vi "FGV Grenzwerte PNS.vi"(0 "Grenzwerte PNS":T5={"Filter:"={"Sollwert"=0.0, "Warn-Min"=0.0, "Warn-Max"=0.0, "Abschalt-Min"=0.0, "Abschalt-Max"=0.0, "Regler"=1, "AnlagenParameter"=""}, "Ventilplatte:"={"Sollwert"=0.0, "Warn-Min"=0.0, "Warn-Max"=0.0, "Abschalt-Min"=0.0, "Abschalt-Max"=0.0, "Regler"=1, "AnlagenParameter"=""}, "Heizleitung 1:"={"Sollwert"=0.0, "Warn-Min"=0.0, "Warn-Max"=0.0, "Abschalt-Min"=0.0, "Abschalt-Max"=0.0, "Regler"=1, "AnlagenParameter"=""}, "Heizleitung 2:"={"Sollwert"=0.0, "Warn-Min"=0.0, "Warn-Max"=0.0, "Abschalt-Min"=0.0, "Abschalt-Max"=0.0, "Regler"=1, "AnlagenParameter"=""}, "Heizleitung 3:"={"Sollwert"=0.0, "Warn-Min"=0.0, "Warn-Max"=0.0, "Abschalt-Min"=0.0, "Abschalt-Max"=0.0, "Regler"=1, "AnlagenParameter"=""}, "Heizleitung 4:"={"Sollwert"=0.0, "Warn-Min"=0.0, "Warn-Max"=0.0, "Abschalt-Min"=0.0, "Abschalt-Max"=0.0, "Regler"=1, "AnlagenParameter"=""}, "Heizleitung 5:"={"Sollwert"=0.0, "Warn-Min"=0.0, "Warn-Max"=0.0, "Abschalt-Min"=0.0, "Abschalt-Max"=0.0, "Regler"=1, "AnlagenParameter"=""}, "Heizleitung 6:"={"Sollwert"=0.0, "Warn-Min"=0.0, "Warn-Max"=0.0, "Abschalt-Min"=0.0, "Abschalt-Max"=0.0, "Regler"=1, "AnlagenParameter"=""}} {"Heizleitung 6:"."Regler" items=["aktiv", "inaktiv"]; "Heizleitung 6:"."Abschalt-Max" format="%#_5g"; "Heizleitung 6:"."Abschalt-Min" format="%#_5g"; "Heizleitung 6:"."Warn-Max" format="%#_5g"; "Heizleitung 6:"."Warn-Min" format="%#_5g"; "Heizleitung 6:"."Sollwert" format="%#_5g"; "Heizleitung 5:"."Regler" items=["aktiv", "inaktiv"]; "Heizleitung 5:"."Abschalt-Max" format="%#_5g"; "Heizleitung 5:"."Abschalt-Min" format="%#_5g"; "Heizleitung 5:"."Warn-Max" format="%#_5g"; "Heizleitung 5:"."Warn-Min" format="%#_5g"; "Heizleitung 5:"."Sollwert" format="%#_5g"; "Heizleitung 4:"."Regler" items=["aktiv", "inaktiv"]; "Heizleitung 4:"."Abschalt-Max" format="%#_5g"; "Heizleitung 4:"."Abschalt-Min" format="%#_5g"; "Heizleitung 4:"."Warn-Max" format="%#_5g"; "Heizleitung 4:"."Warn-Min" format="%#_5g"; "Heizleitung 4:"."Sollwert" format="%#_5g"; "Heizleitung 3:"."Regler" items=["aktiv", "inaktiv"]; "Heizleitung 3:"."Abschalt-Max" format="%#_5g"; "Heizleitung 3:"."Abschalt-Min" format="%#_5g"; "Heizleitung 3:"."Warn-Max" format="%#_5g"; "Heizleitung 3:"."Warn-Min" format="%#_5g"; "Heizleitung 3:"."Sollwert" format="%#_5g"; "Heizleitung 2:"."Regler" items=["aktiv", "inaktiv"]; "Heizleitung 2:"."Abschalt-Max" format="%#_5g"; "Heizleitung 2:"."Abschalt-Min" format="%#_5g"; "Heizleitung 2:"."Warn-Max" format="%#_5g"; "Heizleitung 2:"."Warn-Min" format="%#_5g"; "Heizleitung 2:"."Sollwert" format="%#_5g"; "Heizleitung 1:"."Regler" items=["aktiv", "inaktiv"]; "Heizleitung 1:"."Abschalt-Max" format="%#_5g"; "Heizleitung 1:"."Abschalt-Min" format="%#_5g"; "Heizleitung 1:"."Warn-Max" format="%#_5g"; "Heizleitung 1:"."Warn-Min" format="%#_5g"; "Heizleitung 1:"."Sollwert" format="%#_5g"; "Ventilplatte:"."Regler" items=["aktiv", "inaktiv"]; "Ventilplatte:"."Abschalt-Max" format="%#_5g"; "Ventilplatte:"."Abschalt-Min" format="%#_5g"; "Ventilplatte:"."Warn-Max" format="%#_5g"; "Ventilplatte:"."Warn-Min" format="%#_5g"; "Ventilplatte:"."Sollwert" format="%#_5g"; "Filter:"."Regler" items=["aktiv", "inaktiv"]; "Filter:"."Abschalt-Max" format="%#_5g"; "Filter:"."Abschalt-Min" format="%#_5g"; "Filter:"."Warn-Max" format="%#_5g"; "Filter:"."Warn-Min" format="%#_5g"; "Filter:"."Sollwert" format="%#_5g"}, 1 "T90":bool, 2 "T90 lüften":bool, 5 "IP-Adresse":string, 7 "Anweisungscode":u16, 9 "Zustand":T1, 11 "Samplepoint":u16=1, 12 "Aktionen FGV Grenzwerte":T7) -> (4 "Grenzwerte PNS 2":T2={"Filter:"={"Sollwert"=0.0, "Warn-Min"=0.0, "Warn-Max"=0.0, "Abschalt-Min"=0.0, "Abschalt-Max"=0.0, "Regler"=1, "AnlagenParameter"=""}, "Ventilplatte:"={"Sollwert"=0.0, "Warn-Min"=0.0, "Warn-Max"=0.0, "Abschalt-Min"=0.0, "Abschalt-Max"=0.0, "Regler"=1, "AnlagenParameter"=""}, "Heizleitung 1:"={"Sollwert"=0.0, "Warn-Min"=0.0, "Warn-Max"=0.0, "Abschalt-Min"=0.0, "Abschalt-Max"=0.0, "Regler"=1, "AnlagenParameter"=""}, "Heizleitung 2:"={"Sollwert"=0.0, "Warn-Min"=0.0, "Warn-Max"=0.0, "Abschalt-Min"=0.0, "Abschalt-Max"=0.0, "Regler"=1, "AnlagenParameter"=""}, "Heizleitung 3:"={"Sollwert"=0.0, "Warn-Min"=0.0, "Warn-Max"=0.0, "Abschalt-Min"=0.0, "Abschalt-Max"=0.0, "Regler"=1, "AnlagenParameter"=""}, "Heizleitung 4:"={"Sollwert"=0.0, "Warn-Min"=0.0, "Warn-Max"=0.0, "Abschalt-Min"=0.0, "Abschalt-Max"=0.0, "Regler"=1, "AnlagenParameter"=""}, "Heizleitung 5:"={"Sollwert"=0.0, "Warn-Min"=0.0, "Warn-Max"=0.0, "Abschalt-Min"=0.0, "Abschalt-Max"=0.0, "Regler"=1, "AnlagenParameter"=""}, "Heizleitung 6:"={"Sollwert"=0.0, "Warn-Min"=0.0, "Warn-Max"=0.0, "Abschalt-Min"=0.0, "Abschalt-Max"=0.0, "Regler"=1, "AnlagenParameter"=""}} {"Heizleitung 6:"."Regler" items=["aktiv", "inaktiv"]; "Heizleitung 6:"."Abschalt-Max" format="%#_5g"; "Heizleitung 6:"."Abschalt-Min" format="%#_5g"; "Heizleitung 6:"."Warn-Max" format="%#_5g"; "Heizleitung 6:"."Warn-Min" format="%#_5g"; "Heizleitung 6:"."Sollwert" format="%#_5g"; "Heizleitung 5:"."Regler" items=["aktiv", "inaktiv"]; "Heizleitung 5:"."Abschalt-Max" format="%#_5g"; "Heizleitung 5:"."Abschalt-Min" format="%#_5g"; "Heizleitung 5:"."Warn-Max" format="%#_5g"; "Heizleitung 5:"."Warn-Min" format="%#_5g"; "Heizleitung 5:"."Sollwert" format="%#_5g"; "Heizleitung 4:"."Regler" items=["aktiv", "inaktiv"]; "Heizleitung 4:"."Abschalt-Max" format="%#_5g"; "Heizleitung 4:"."Abschalt-Min" format="%#_5g"; "Heizleitung 4:"."Warn-Max" format="%#_5g"; "Heizleitung 4:"."Warn-Min" format="%#_5g"; "Heizleitung 4:"."Sollwert" format="%#_5g"; "Heizleitung 3:"."Regler" items=["aktiv", "inaktiv"]; "Heizleitung 3:"."Abschalt-Max" format="%#_5g"; "Heizleitung 3:"."Abschalt-Min" format="%#_5g"; "Heizleitung 3:"."Warn-Max" format="%#_5g"; "Heizleitung 3:"."Warn-Min" format="%#_5g"; "Heizleitung 3:"."Sollwert" format="%#_5g"; "Heizleitung 2:"."Regler" items=["aktiv", "inaktiv"]; "Heizleitung 2:"."Abschalt-Max" format="%#_5g"; "Heizleitung 2:"."Abschalt-Min" format="%#_5g"; "Heizleitung 2:"."Warn-Max" format="%#_5g"; "Heizleitung 2:"."Warn-Min" format="%#_5g"; "Heizleitung 2:"."Sollwert" format="%#_5g"; "Heizleitung 1:"."Regler" items=["aktiv", "inaktiv"]; "Heizleitung 1:"."Abschalt-Max" format="%#_5g"; "Heizleitung 1:"."Abschalt-Min" format="%#_5g"; "Heizleitung 1:"."Warn-Max" format="%#_5g"; "Heizleitung 1:"."Warn-Min" format="%#_5g"; "Heizleitung 1:"."Sollwert" format="%#_5g"; "Ventilplatte:"."Regler" items=["aktiv", "inaktiv"]; "Ventilplatte:"."Abschalt-Max" format="%#_5g"; "Ventilplatte:"."Abschalt-Min" format="%#_5g"; "Ventilplatte:"."Warn-Max" format="%#_5g"; "Ventilplatte:"."Warn-Min" format="%#_5g"; "Ventilplatte:"."Sollwert" format="%#_5g"; "Filter:"."Regler" items=["aktiv", "inaktiv"]; "Filter:"."Abschalt-Max" format="%#_5g"; "Filter:"."Abschalt-Min" format="%#_5g"; "Filter:"."Warn-Max" format="%#_5g"; "Filter:"."Warn-Min" format="%#_5g"; "Filter:"."Sollwert" format="%#_5g"}, 6 "IP-Adresse":string, 15 "Anweisungscode":u16)   [LabVIEW 2020, in "PNS.lvlib"]
uses:
  PNS.lvlib
  Aktionen FGV Grenzwerte.ctl
  Anlagengrenzwerte PNS.ctl
  Anlagengrenzwerte-Parameter Anzeige.ctl
  Visualisierungs Elemente/Zahlen-Eingabefeld.ctl
  ObjektKlassen/Steuerung PNS/Anlegengrenzwerte PNS.ctl
  ObjektKlassen/Steuerung PNS/Anlagengrenzwerte Parameteranzeige.ctl
  Funktionstasten/Zustaende.ctl
  Seiten/System Einstellungen V2/Aktioen FGV System.ctl
  Seiten/Erweiterte Konfig/FGV PID Aktionen.ctl
  Seiten/CalGas Aufschaltung/FGV CalGas Aktionen.ctl
  Seiten/System Einstellungen V2/System Einstellungen V2.lvlib
  Seiten/Erweiterte Konfig/Erweiterte Konfig.lvlib
  Seiten/CalGas Aufschaltung/CalGas Aufschaltung.lvlib
  Allgemein/allgemeine Sub-VIs.lvlib
  Funktionstasten/Funktionstasten.lvlib
  ObjektKlassen/Steuerung PNS/Steuerung PNS.lvclass
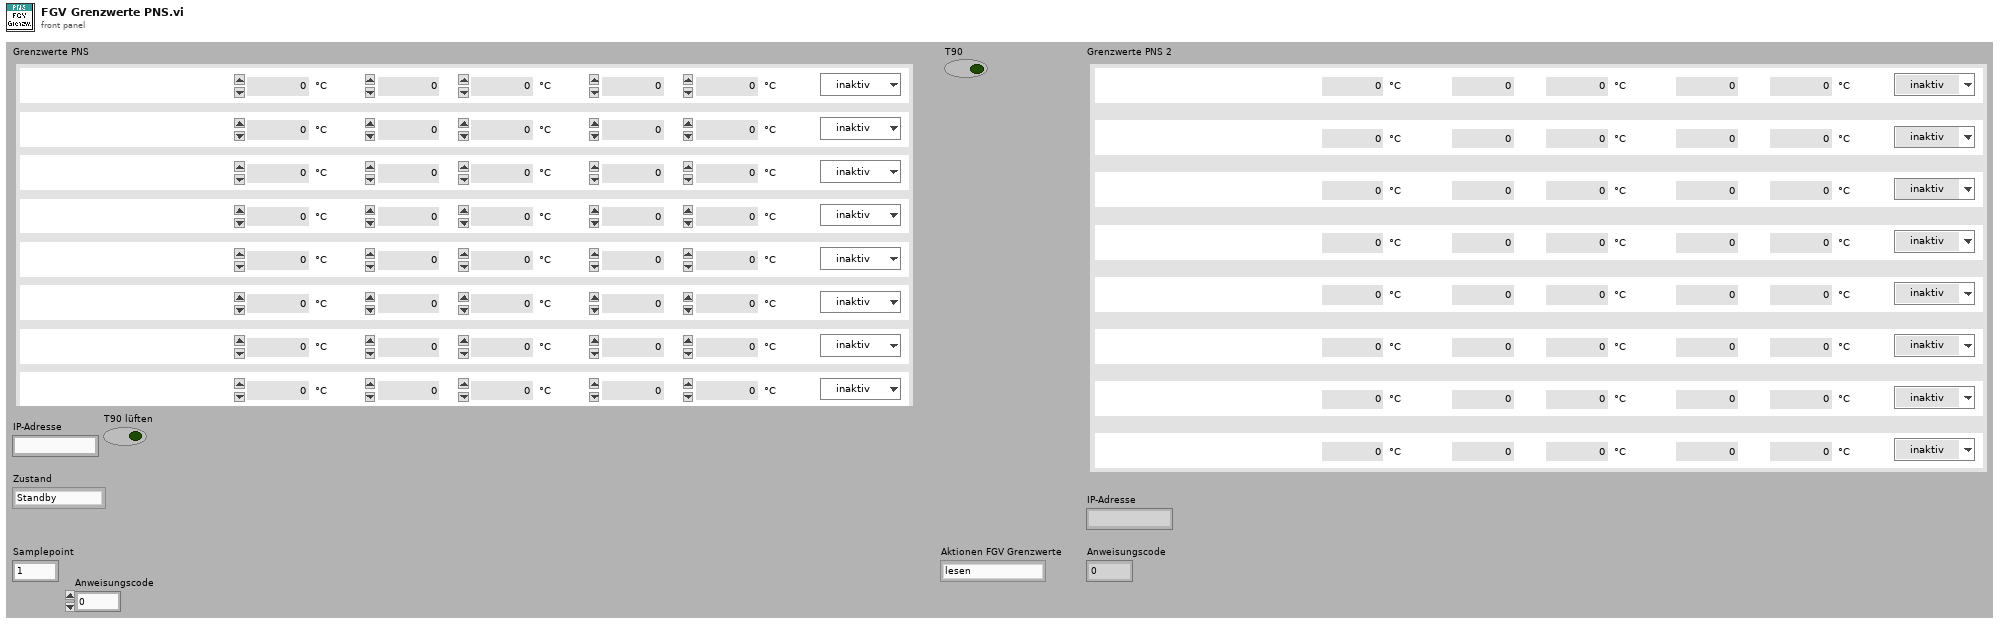
[diagram p1: front panel]
types:
  T1 = typedef "Funktionstasten.lvlib/Zustaende.ctl" = enum16{"Standby", "Pause", "Eco", "Messen", "Kalibrieren", "Spülen Filter", "Spülen Leitung", "Umgebungsluft", "0-Gas", "Cal-Gas", "CG zu PNS", "-------------", "Init 1", "Init 2", "Init 3", "Init 4", "Messen vorbereiten", "Messen durchführen", "Exit"}
  T2 = typedef "Steuerung PNS.lvclass/Anlegengrenzwerte PNS.ctl" = cluster{"Filter:":T3, "Ventilplatte:":T3, "Heizleitung 1:":T3, "Heizleitung 2:":T3, "Heizleitung 3:":T3, "Heizleitung 4:":T3, "Heizleitung 5:":T3, "Heizleitung 6:":T3}
  T3 = typedef "Steuerung PNS.lvclass/Anlagengrenzwerte Parameteranzeige.ctl" = cluster{"Sollwert":T4, "Warn-Min":T4, "Warn-Max":T4, "Abschalt-Min":T4, "Abschalt-Max":T4, "Regler":u16, "AnlagenParameter":string}
  T4 = typedef "Zahlen-Eingabefeld.ctl" = sgl
  T5 = typedef "PNS.lvlib/Anlagengrenzwerte PNS.ctl" = cluster{"Filter:":T6, "Ventilplatte:":T6, "Heizleitung 1:":T6, "Heizleitung 2:":T6, "Heizleitung 3:":T6, "Heizleitung 4:":T6, "Heizleitung 5:":T6, "Heizleitung 6:":T6}
  T6 = typedef "PNS.lvlib/Anlagengrenzwerte-Parameter Anzeige.ctl" = cluster{"Sollwert":T4, "Warn-Min":T4, "Warn-Max":T4, "Abschalt-Min":T4, "Abschalt-Max":T4, "Regler":u16, "AnlagenParameter":string}
  T7 = typedef "PNS.lvlib/Aktionen FGV Grenzwerte.ctl" = enum16{"lesen", "Grenzw. schreiben", "Anweisungscode", "IP-Adresse", "laden", "speichern", "Anweisungscode vorgeben"}
  T8 = typedef "Erweiterte Konfig.lvlib/FGV PID Aktionen.ctl" = enum16{"Lesen", "Schreiben PID", "Schreiben Sonstige", "Dichtheitstest", "Aktionen Dicht.", "Parameter Sensor"}
  T9 = typedef "System Einstellungen V2.lvlib/Aktioen FGV System.ctl" = enum16{"lesen", "laden", "speichern", "Optionen schreiben", "Zeitstempel", "Reset BMP", "Reset SQP", "Wartung", "Werkseinstellung"}
  T10 = typedef "CalGas Aufschaltung.lvlib/FGV CalGas Aktionen.ctl" = enum16{"lesen", "Analysator Auswahl", "Def.CalGas", "Aufschaltung CalGas", "laden", "speichern", "KAL extrahieren"}
  T11 = typedef "System Einstellungen.lvlib/Optionen.ctl" = cluster{"Störmeldep.":bool, "Betriebszustände":bool, "LN2 Befüllung":bool, "Klimaanlage ?":bool, "AK in ppm":bool, "log Cal-Gas":bool, "log 0-Gas":bool, "log CG zu PNS":bool, "Reserve":bool, "Reserve1":bool, "PNS?":bool, "Container":bool, "Mit N2 spülen":bool, "Span Gas Auswahl":T12}
  T12 = typedef "Funktionstasten.lvlib/Spaneingang.ctl" = u16
  T13 = typedef "System Einstellungen V2.lvlib/Optionen.ctl" = cluster{"Störmeldep.":bool, "Betriebszustände":bool, "AK in ppm":bool, "log Cal-Gas":bool, "log 0-Gas":bool, "Durchflusssensor 0-5V":bool, "PNS?":bool, "Mit N2 spülen":bool, "TRE08":bool, "Amium 10-Fach":bool, "Verticale Scrollbar aktiv":bool, "Loggingtakt":bool, "AK Rezeptwechsel gleich wie MKS":bool, "NG ECO":bool}
  T14 = typedef "CalGas Aufschaltung.lvlib/Aufschaltung CalGas.ctl" = cluster{"Kalibriergas":T15, "Aufschaltpunkt":T16, "Analysator":T17}
  T15 = typedef "Auswahlfeld.ctl" = u16
  T16 = typedef "CalGas Aufschaltung.lvlib/Auswahl Aufschaltpunkt.ctl" = enum16{"über Filterblock", "Analysator direkt", "über PNS", "Entnahme"}
  T17 = typedef "CalGas Aufschaltung.lvlib/Auswahl Analysator.ctl" = enum16{"FT-IR", "FID", "PMA", "PMA/FID/FT-IR"}
  T18 = cluster{"Grenzwerte PNS":T5, "IP-Adresse":string}
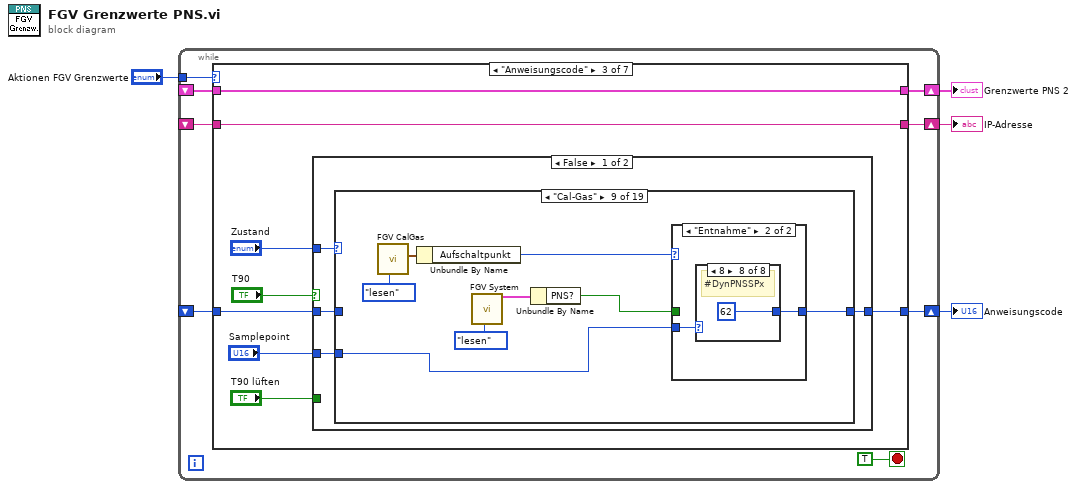
[diagram p0: block diagram]
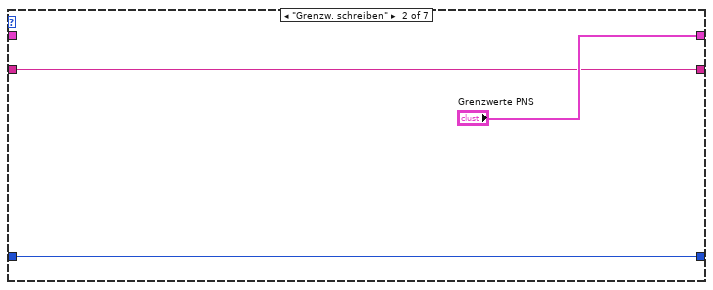
[diagram p3: hidden frame]
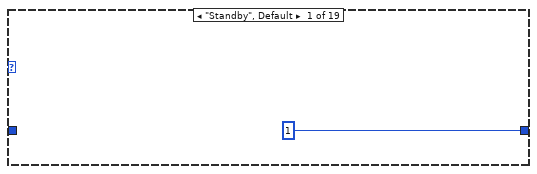
[diagram p4: hidden frame]
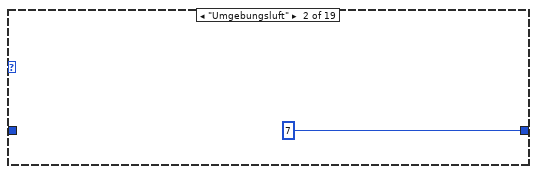
[diagram p5: hidden frame]
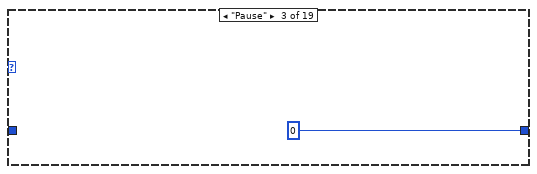
[diagram p6: hidden frame]
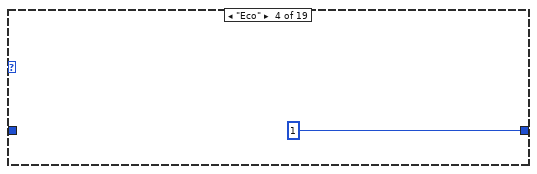
[diagram p7: hidden frame]
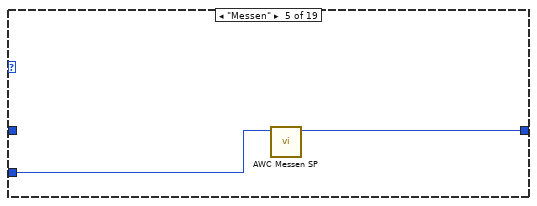
[diagram p8: hidden frame]
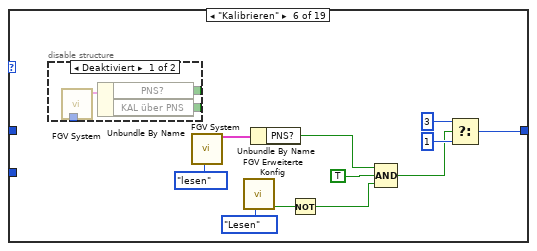
[diagram p9: hidden frame]
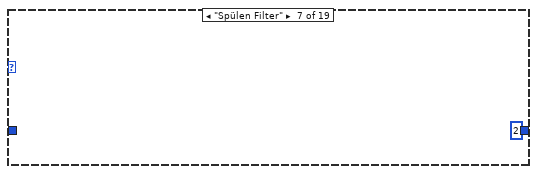
[diagram p11: hidden frame]
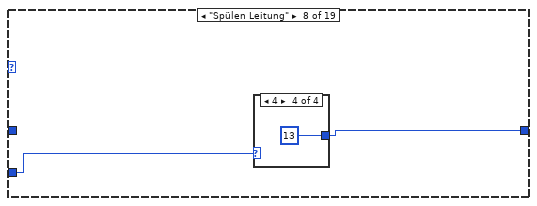
[diagram p12: hidden frame]
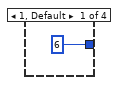
[diagram p13: hidden frame]
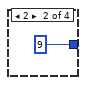
[diagram p14: hidden frame]
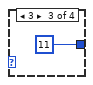
[diagram p15: hidden frame]
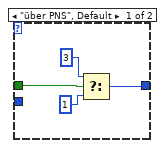
[diagram p16: hidden frame]
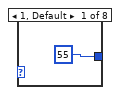
[diagram p17: hidden frame]
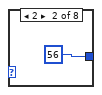
[diagram p18: hidden frame]
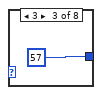
[diagram p19: hidden frame]
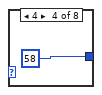
[diagram p20: hidden frame]
diagram:
  n1 = while {
    tunnel: "Aktionen FGV Grenzwerte" -> [w11]
    shift-right: [w10] -> w3
    shift-left: _ -> [w9]
    shift-right: [w7] -> w2
    shift-left: _ -> [w8]
    shift-right: [w6] -> w1
    shift-left: _ -> [w5]
    stop <- TRUE stop-if-true
    n2 = case shown="\"Anweisungscode\"" w11 {
      tunnel: [w15 "Grenzwerte PNS" w26 w142 w149 w199 w203] -> w10
      tunnel: w9 -> [w15 _ w26 w142 w158 w199 w203]
      tunnel: w8 -> [w13 w17 w21 w141 w162 w200 _]
      tunnel: [w13 w17 w25 w141 w162 w200 "Anweisungscode"] -> w7
      tunnel: [w14 w16 w24 "IP-Adresse" w145 w198 w202] -> w6
      tunnel: w5 -> [w14 w16 w24 _ w157 w198 w202]
      frame "lesen", Default {
      }
      frame "Grenzw. schreiben" {
      }
      frame "Anweisungscode" {
        n3 = case shown="False" "T90" {
          tunnel: [w30 w137] -> w25
          tunnel: "Zustand" -> [w29 _]
          tunnel: "Samplepoint" -> [w28 w135]
          tunnel: w21 -> [w27 _]
          tunnel: "T90 lüften" -> [_ w136]
          frame False {
            n4 = case shown="\"Cal-Gas\"" w29 {
              tunnel: [u16 1 ("Anweisungscode") u16 7 ("Anweisungscode") u16 0 ("Anweisungscode") u16 1 ("Anweisungscode") w36 w46 u16 2 ("Anweisungscode") w53 w64 w86 w108 u16 1 ("Anweisungscode") u16 1 ("Anweisungscode") u16 1 ("Anweisungscode") u16 1 ("Anweisungscode") u16 1 ("Anweisungscode") w130 w132 u16 1 ("Anweisungscode")] -> w30
              tunnel: w28 -> [_ _ _ _ w35 _ _ w54 w59 w81 w103 _ _ _ _ _ w131 w133 _]
              tunnel: w27 -> [_ _ _ _ _ _ _ _ _ _ _ _ _ _ _ _ _ _ _]
              frame "Standby", Default {
              }
              frame "Umgebungsluft" {
              }
              frame "Pause" {
              }
              frame "Eco" {
              }
              frame "Messen" {
                n5 = call "AWC Messen SP.vi"("Samplepoint"=w35) -> ("Anweisungscode"=w36:u16)  [unwired: 10 in]
              }
              frame "Kalibrieren" {
                n6 = disable-structure shown="Deaktiviert" {
                  disable-tunnel: _ -> [w51 _]
                  disable-tunnel: [w49 _] -> _
                  disable-tunnel: [w48 _] -> _
                  frame Disabled {
                    n7 = call "FGV System.vi"("Aktionen"=w51) -> ("Optionen"=w50:T11)  [unwired: 8 in, 2 out]
                    n8 = Unbundle By Name(w50) -> ("PNS?"=w49:bool, "KAL über PNS"=w48:bool)
                  }
                  frame Enabled {
                  }
                }
                n9 = call "FGV System.vi"("Aktionen"=Aktioen_FGV_System."lesen") -> ("Optionen"=w38:T13)  [unwired: 12 in, 6 out]
                n10 = call "FGV Erweiterte Konfig.vi"("Aktion"=FGV_PID_Aktionen."Lesen") -> ("Dichtheitstest?"=w44:bool)  [unwired: 6 in, 4 out]
                n11 = Unbundle By Name(w38) -> ("PNS?"=w43:bool)
                n12 = Not(x=w44) -> (.not. x?=w42:bool)
                n13 = Compound Arithmetic op=AND(w43, TRUE ("Wert"), w42) -> (w39:bool)
                n14 = Select(t=u16 3 ("Anweisungscode"), s=w39, f=u16 1 ("Anweisungscode")) -> (s? t:f=w46:u16)
              }
              frame "Spülen Filter" {
                # "#PNStakten"
              }
              frame "Spülen Leitung" {
                n15 = case shown="4" w54 {
                  tunnel: [u16 6 ("Anweisungscode") u16 9 ("Anweisungscode") u16 11 ("Anweisungscode") u16 13 ("Anweisungscode")] -> w53
                  frame 1, Default {
                  }
                  frame 2 {
                  }
                  frame 3 {
                  }
                  frame 4 {
                  }
                }
              }
              frame "Cal-Gas" {
                n16 = call "FGV CalGas.vi"("Aktionen"=FGV_CalGas_Aktionen."lesen") -> ("Aufschaltung CalGas"=w65:T14)  [unwired: 6 in, 4 out]
                n17 = Unbundle By Name(w65) -> ("Aufschaltpunkt"=w61:T16)
                n18 = call "FGV System.vi"("Aktionen"=Aktioen_FGV_System."lesen") -> ("Optionen"=w63:T13)  [unwired: 12 in, 6 out]
                n19 = Unbundle By Name(w63) -> ("PNS?"=w60:bool)
                n20 = case shown="\"Entnahme\"" w61 {
                  tunnel: [w69 w72] -> w64
                  tunnel: w60 -> [w68 _]
                  tunnel: w59 -> [_ w71]
                  frame "über PNS", Default {
                    n21 = Select(t=u16 3 ("Anweisungscode"), s=w68, f=u16 1 ("Anweisungscode")) -> (s? t:f=w69:u16)
                  }
                  frame "Entnahme" {
                    n22 = case shown="8" w71 {
                      tunnel: [u16 55 ("Anweisungscode") u16 56 ("Anweisungscode") u16 57 ("Anweisungscode") u16 58 ("Anweisungscode") u16 59 ("Anweisungscode") u16 60 ("Anweisungscode") u16 61 ("Anweisungscode") u16 62 ("Anweisungscode")] -> w72
                      frame 1, Default {
                      }
                      frame 2 {
                      }
                      frame 3 {
                      }
                      frame 4 {
                      }
                      frame 5 {
                      }
                      frame 6 {
                      }
                      frame 7 {
                      }
                      frame 8 {
                        # "#DynPNSSPx"
                      }
                    }
                  }
                }
              }
              frame "0-Gas" {
                n23 = call "FGV CalGas.vi"("Aktionen"=FGV_CalGas_Aktionen."lesen") -> ("Aufschaltung CalGas"=w87:T14)  [unwired: 6 in, 4 out]
                n24 = call "FGV System.vi"("Aktionen"=Aktioen_FGV_System."lesen") -> ("Optionen"=w85:T13)  [unwired: 12 in, 6 out]
                n25 = Unbundle By Name(w87) -> ("Aufschaltpunkt"=w83:T16)
                n26 = Unbundle By Name(w85) -> ("PNS?"=w82:bool)
                n27 = case shown="\"über PNS\", Standard" w83 {
                  tunnel: [w91 w94] -> w86
                  tunnel: w82 -> [w90 _]
                  tunnel: w81 -> [_ w93]
                  frame "über PNS", Default {
                    n28 = Select(t=u16 3 ("Anweisungscode"), s=w90, f=u16 1 ("Anweisungscode")) -> (s? t:f=w91:u16)
                  }
                  frame "Entnahme" {
                    n29 = case shown="8" w93 {
                      tunnel: [u16 55 ("Anweisungscode") u16 56 ("Anweisungscode") u16 57 ("Anweisungscode") u16 58 ("Anweisungscode") u16 59 ("Anweisungscode") u16 60 ("Anweisungscode") u16 61 ("Anweisungscode") u16 62 ("Anweisungscode")] -> w94
                      frame 1, Default {
                      }
                      frame 2 {
                      }
                      frame 3 {
                      }
                      frame 4 {
                      }
                      frame 5 {
                      }
                      frame 6 {
                      }
                      frame 7 {
                      }
                      frame 8 {
                        # "#DynPNSSPx"
                      }
                    }
                  }
                }
              }
              frame "CG zu PNS" {
                n30 = call "FGV CalGas.vi"("Aktionen"=FGV_CalGas_Aktionen."lesen") -> ("Aufschaltung CalGas"=w109:T14)  [unwired: 6 in, 4 out]
                n31 = call "FGV System.vi"("Aktionen"=Aktioen_FGV_System."lesen") -> ("Optionen"=w107:T13)  [unwired: 12 in, 6 out]
                n32 = Unbundle By Name(w109) -> ("Aufschaltpunkt"=w105:T16)
                n33 = Unbundle By Name(w107) -> ("PNS?"=w104:bool)
                n34 = case shown="\"Entnahme\"" w105 {
                  tunnel: [w113 w116] -> w108
                  tunnel: w104 -> [w112 _]
                  tunnel: w103 -> [_ w115]
                  frame "über PNS", Default {
                    n35 = Select(t=u16 3 ("Anweisungscode"), s=w112, f=u16 1 ("Anweisungscode")) -> (s? t:f=w113:u16)
                  }
                  frame "Entnahme" {
                    n36 = case shown="5" w115 {
                      tunnel: [u16 55 ("Anweisungscode") u16 56 ("Anweisungscode") u16 57 ("Anweisungscode") u16 58 ("Anweisungscode") u16 59 ("Anweisungscode") u16 60 ("Anweisungscode") u16 61 ("Anweisungscode") u16 62 ("Anweisungscode")] -> w116
                      frame 1, Default {
                      }
                      frame 2 {
                      }
                      frame 3 {
                      }
                      frame 4 {
                      }
                      frame 5 {
                      }
                      frame 6 {
                      }
                      frame 7 {
                      }
                      frame 8 {
                        # "#DynPNSSPx"
                      }
                    }
                  }
                }
              }
              frame "-------------" {
              }
              frame "Init 1" {
              }
              frame "Init 2" {
              }
              frame "Init 3" {
              }
              frame "Init 4" {
              }
              frame "Messen vorbereiten" {
                n37 = call "AWC Messen SP.vi"("Samplepoint"=w131) -> ("Anweisungscode"=w130:u16)  [unwired: 10 in]
              }
              frame "Messen durchführen" {
                n38 = call "AWC Messen SP.vi"("Samplepoint"=w133) -> ("Anweisungscode"=w132:u16)  [unwired: 10 in]
              }
              frame "Exit" {
              }
            }
          }
          frame True {
            # "#T90LP"
            n39 = case shown="False" w136 {
              tunnel: [w138 u16 7 ("Anweisungscode")] -> w137
              tunnel: w135 -> [w139 _]
              frame False {
                n40 = call "AWC T90.vi"("Samplepoint"=w139) -> ("Anweisungscode"=w138:u16)  [unwired: 10 in]
              }
              frame True {
              }
            }
          }
        }
      }
      frame "IP-Adresse" {
      }
      frame "laden" {
        w152 = "Config_PNS.bin" ("Dateiname")
        n41 = call "Datei im Ordner des VI (EXE).vi"("Dateiname"=w152) -> ("Ordner des Haupt-VIs"=w153:path, "Dateipfad im Ordner des Haupt-VIs"=w161:path)  [unwired: 8 in, 1 out]
        n42 = Bundle("Grenzwerte PNS"=w158, "IP-Adresse"=w157) -> (w159:T18)  [unwired: 1 in]
        n43 = Open/Create/Replace File(file path (use dialog)=w161) -> (refnum out=w160:refnum<file>, error out=w144:errorcluster)  [unwired: 5 in, 1 out]
        n44 = Read from Binary File(5:w159, 8:w144, 11:w160) -> (0:w155:errorcluster, 2:w156:T18, 3:w154:refnum<file>)  [unwired: 1 in, 3 out]
        n45 = case shown="Fehler" w155 {
          selector: w155 -> [w165 w169]
          tunnel: w153 -> [_ w170]
          tunnel: w156 -> [w166 w168]
          tunnel: [w166 w176] -> w150
          tunnel: [w163 w174] -> w151
          tunnel: w154 -> [w164 _]
          tunnel: w152 -> [_ w167]
          frame No Error {
            n46 = Close File(refnum=w164, error in=w165) -> (error out=w163:errorcluster)  [unwired: 1 out]
          }
          frame Error {
            n47 = call "Factorysettings Pfad.vi"("error in (no error)"=w169, "Dateiname"=w167, "Ordner des Haupt-VIs"=w170) -> ("error out"=w171:errorcluster, "Pfad Factorysettings"=w172:path)  [unwired: 7 in]
            n48 = for {
              N: 3 -> [_]
              tunnel: w171 -> [w183]
              tunnel: w172 -> [w182]
              tunnel: [w181] -> w176
              tunnel: [w180] -> w175
              tunnel: [w179] -> w173
              tunnel: w168 -> [w178]
              stop <- w184 stop-if-true
              n49 = Read from Binary File(5:w178, 8:w183, 11:w182) -> (0:w185:errorcluster, 2:w181:T18, 3:w179:refnum<file>)  [unwired: 3 in, 1 out]
              n50 = case shown="Kein Fehler" w185 {
                selector: w185 -> [_ w188]
                tunnel: [TRUE _] -> w184
                tunnel: [errorcluster {"status"=FALSE, "code"=0, "source"=""} ("error IO") w188] -> w180
                frame No Error {
                }
                frame Error {
                  n51 = Wait (ms)(milliseconds to wait=u32 100 ("Zu wartende ms")) -> ()  [unwired: 1 out]
                }
              }
            }
            n52 = Close File(refnum=w173, error in=w175) -> (error out=w174:errorcluster)  [unwired: 1 out]
          }
        }
        n53 = call <vilib>:"Clear Errors.vi"("error in (no error)"=w151) -> ()  [unwired: 5 in, 2 out]
        n54 = Unbundle(w150) -> ("Grenzwerte PNS"=w149:T5, "IP-Adresse"=w146:string)
        n55 = Empty String/Path?(string/path=w146) -> (empty?=w148:bool)
        n56 = Select(t="192.168.15.101" ("IP-Adresse"), s=w148, f=w146) -> (s? t:f=w145:string)
      }
      frame "speichern" {
        n57 = Bundle("Grenzwerte PNS"=w199, "IP-Adresse"=w198) -> (w193:T18)  [unwired: 1 in]
        n58 = call "Datei im Ordner des VI (EXE).vi"("Dateiname"="Config_PNS.bin") -> ("Dateipfad im Ordner des Haupt-VIs"=w197:path)  [unwired: 8 in, 2 out]
        n59 = Open/Create/Replace File(file path (use dialog)=w197) -> (refnum out=w195:refnum<file>, error out=w194:errorcluster)  [unwired: 5 in, 1 out]
        n60 = Write to Binary File(file (use dialog)=w195, data=w193, error in=w194) -> (refnum out=w191:refnum<file>, error out=w192:errorcluster)  [unwired: 4 out]
        n61 = Close File(refnum=w191, error in=w192) -> (error out=w190:errorcluster)  [unwired: 1 out]
        n62 = call <vilib>:"Clear Errors.vi"("error in (no error)"=w190) -> ()  [unwired: 5 in, 2 out]
      }
      frame "Anweisungscode vorgeben" {
      }
    }
  }
  "Grenzwerte PNS 2" <- w3
  "Anweisungscode" <- w2
  "IP-Adresse" <- w1
